vi "Split Registers by Direction.vi"(7 "Group":bool, 8 "error in":errorcluster, 11 "vi info":T2 {"RegisterMap"."Address" format="%.0x"}) -> (0 "error out":errorcluster, 1 "FXP channels out":T1(array[cluster]), 2 "Controls":T9[](array[typedef]) {"Data Type" format="%.0x"}, 3 "Indicator":T9[](array[typedef]) {"Data Type" format="%.0x"})   [LabVIEW 2018, in "FPGA Addon System Explorer.lvlib"]
uses:
  FPGA Addon System Explorer.lvlib
  Addon Shared/Types/Register Information.ctl
  Addon Shared/Types/Data Type.ctl
  <vilib>/rvi/Bitfile/niFpgaBitfileStructure_VI.ctl
  <vilib>/rvi/Bitfile/nirviControlStructure.ctl
  <vilib>/rvi/Bitfile/nirviTypdefDescription.ctl
  <vilib>/rvi/Bitfile/nirviMechanicalAction.ctl
  <vilib>/rvi/Bitfile/nirviSubControlStructure.ctl
  <vilib>/rvi/Bitfile/nirviClusterElementControl.ctl
  <vilib>/picture/picture.llb/imagedata.ctl
  Submodules/Source/Types/PWM.Measure.Analog.Measurement.ctl
  Submodules/Source/Types/PWM.Measure.Digital.Measurement.ctl
  Submodules/Source/Types/Static.Measure.Digital.Measurement.ctl
  Submodules/Source/Types/QuadratureEncoder.Measure.Digital.Measurement.ctl
  Submodules/Source/Types/PWM.Generate.Digital.Settings.ctl
  Submodules/Source/Types/PWM.Measure.Analog.Settings.ctl
  Submodules/Source/Types/PWM.Measure.Digital.Settings.ctl
  Submodules/Source/Types/Sine.Generate.Settings.ctl
  Submodules/Source/Types/Static.Generate.Digital.Settings.ctl
  Submodules/Source/Types/Static.Measure.Digital.Settings.ctl
  Submodules/Source/Types/WSS.Generate.Digital.Settings.ctl
  Submodules/Source/Types/QuadratureEncoder.Measure.Digital.Settings.ctl
  Addon Shared/FPGA Addon Shared.lvlib
  Submodules/Source/Speciality FPGA IO.lvlib
  <vilib>/Utility/Data Type/NI_Data Type.lvlib
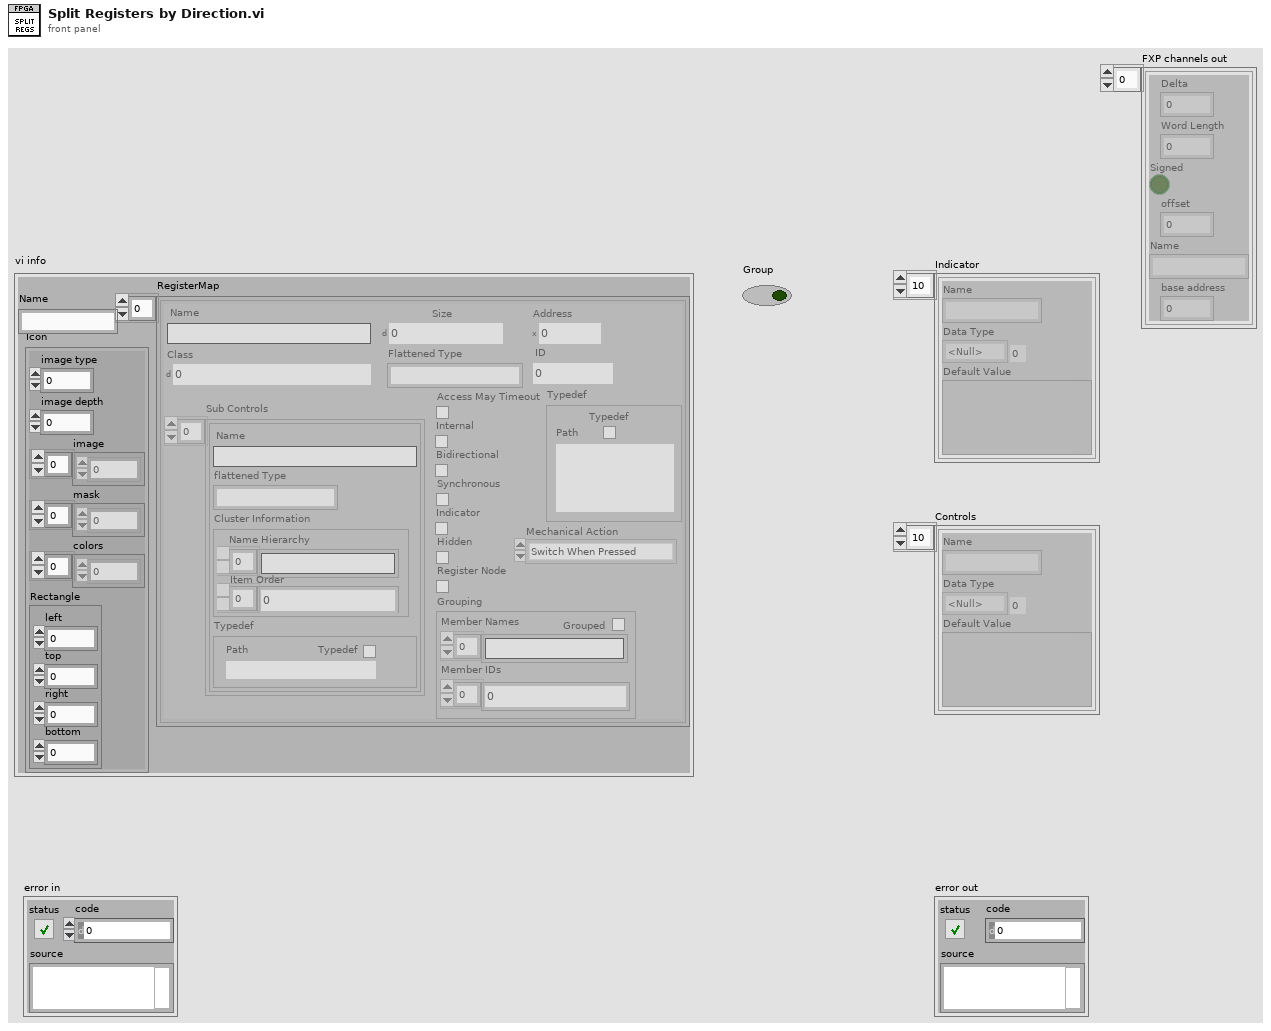
[diagram p1: front panel]
types:
  T1 = cluster{"Delta":dbl, "Word Length":i8, "Signed":bool, "offset":i32, "Name":string, "base address":i32}[]
  T2 = typedef "niFpgaBitfileStructure_VI.ctl" = cluster{"Name":string, "RegisterMap":T3[], "Icon":T8}
  T3 = typedef "nirviControlStructure.ctl" = cluster{"Name":string, "Hidden":bool, "Indicator":bool, "Flattened Type":string, "Grouping":cluster{"Grouped":bool, "Member Names":string[], "Member IDs":u32[]}, "Address":u32, "Size":u32, "Class":u32, "Internal":bool, "Typedef":T4, "ID":u32, "Bidirectional":bool, "Synchronous":bool, "Mechanical Action":T5, "Sub Controls":T6[], "Access May Timeout":bool, "Register Node":bool}
  T4 = typedef "nirviTypdefDescription.ctl" = cluster{"Typedef":bool, "Path":path}
  T5 = typedef "nirviMechanicalAction.ctl" = enum8{"Switch When Pressed", "Switch When Released", "Switch Until Released", "Latch When Pressed", "Latch When Released", "Latch Until Released"}
  T6 = typedef "nirviSubControlStructure.ctl" = cluster{"Name":string, "flattened Type":string, "Cluster Information":T7, "Typedef":T4}
  T7 = typedef "nirviClusterElementControl.ctl" = cluster{"Name Hierarchy":string[], "Item Order":u32[]}
  T8 = typedef "imagedata.ctl" = cluster{"image type":i32, "image depth":i32, "image":u8[], "mask":u8[], "colors":u32[], "Rectangle":cluster{"left":i16, "top":i16, "right":i16, "bottom":i16}}
  T9 = typedef "FPGA Addon Shared.lvlib/Register Information.ctl" = cluster{"Name":string, "Data Type":T10, "Default Value":variant}
  T10 = typedef "FPGA Addon Shared.lvlib/Data Type.ctl" = enum8{"<Null>", "I8", "I16", "I32", "I64", "U8", "U16", "U32", "U64", "SGL", "Boolean", "Analog PWM In Settings", "Analog PWM In", "Digital PWM In Settings", "Digital PWM In", "Digital PWM Out", "Sine Out", "FXP+/-24.5", "FXP+/-16.5", "FXP+/-32.8", "FXP+/-64.32", "FXP+/-16.7", "FXP+/-20.5", "FXP+/-27.5", "FXP+/-32.16", "FXP+16.3", "FXP+18.3", "Digital Static In", "Digital Static Out", "Digital Static In Settings", "Digital WSS Out", "Quad Encoder Settings", "Quad Encoder In", "Group"}
  T11 = typedef "Speciality FPGA IO.lvlib/QuadratureEncoder.Measure.Digital.Measurement.ctl" = cluster{"POSITION":i32}
  T12 = typedef "Speciality FPGA IO.lvlib/Static.Measure.Digital.Measurement.ctl" = cluster{"STATE":bool}
  T13 = typedef "Speciality FPGA IO.lvlib/PWM.Measure.Digital.Measurement.ctl" = cluster{"ACTIVE TICKS":u32, "INACTIVE TICKS":u32, "ACQ TICKS":u32}
  T14 = typedef "Speciality FPGA IO.lvlib/PWM.Measure.Analog.Measurement.ctl" = cluster{"ACTIVE TICKS":u32, "INACTIVE TICKS":u32, "ACQ TICKS":u32, "ACTIVE VOLTAGE":fxp<+/-,32,8>, "INACTIVE VOLTAGE":fxp<+/-,32,8>}
  T15 = typedef "Speciality FPGA IO.lvlib/QuadratureEncoder.Measure.Digital.Settings.ctl" = cluster{"DIRECTION":u8, "RESET VALUE":i32, "A RESET STATE":bool, "B RESET STATE":bool, "Z RESET STATE":bool}
  T16 = typedef "Speciality FPGA IO.lvlib/WSS.Generate.Digital.Settings.ctl" = cluster{"ACTIVE EDGE":bool, "ACTIVE TICKS":u32, "INACTIVE TICKS":u32, "DATA":u8, "SENSOR TYPE":u8}
  T17 = typedef "Speciality FPGA IO.lvlib/Static.Measure.Digital.Settings.ctl" = cluster{"ACTIVE EDGE":bool}
  T18 = typedef "Speciality FPGA IO.lvlib/Static.Generate.Digital.Settings.ctl" = cluster{"ACTIVE EDGE":bool, "OUTPUT":bool}
  T19 = typedef "Speciality FPGA IO.lvlib/Sine.Generate.Settings.ctl" = cluster{"AMP":fxp<+/-,32,8>, "OFFSET":fxp<+/-,32,8>, "PERIODS/TICKS":fxp<+,32,0>}
  T20 = typedef "Speciality FPGA IO.lvlib/PWM.Measure.Digital.Settings.ctl" = cluster{"ACTIVE EDGE":bool, "TIMEOUT":u32}
  T21 = typedef "Speciality FPGA IO.lvlib/PWM.Measure.Analog.Settings.ctl" = cluster{"ACTIVE EDGE":bool, "TIMEOUT":u32, "THRESHOLD":fxp<+/-,32,8>}
  T22 = typedef "Speciality FPGA IO.lvlib/PWM.Generate.Digital.Settings.ctl" = cluster{"ACTIVE EDGE":bool, "ACTIVE TICKS":u32, "INACTIVE TICKS":u32}
  T23 = cluster{"Delta":dbl, "Word Length":i8, "Signed":bool, "offset":i32, "Name":string, "base address":i32}
  T24 = typedef "Type Descriptor Enumeration__ogtk.ctl" = enum8{"<Null>", "I8", "I16", "I32", "I64", "U8", "U16", "U32", "U64", "SGL", "DBL", "EXT", "CSG", "CDB", "CXT", "0x0F", "0x10", "0x11", "0x12", "0x13", "0x14", "Enum U8", "Enum U16", "Enum U32", "Enum U64", "SGL PQ", "DBL PQ", "EXT PQ", "CSG PQ", "CDB PQ", "CXT PQ", "0x1F", "0x20", "Boolean", "0x22", "0x23", "0x24", "0x25", "0x26", "0x27", "0x28", "0x29", "0x2A", "0x2B", "0x2C", "0x2D", "0x2E", "0x2F", "String", "0x31", "Path", "Pict", "0x34", "0x35", "0x36", "DAQ", "0x38", "0x39", "0x3A", "0x3B", "0x3C", "0x3D", "0x3E", "0x3F", "Array", "0x41", "0x42", "0x43", "0x44", "0x45", "0x46", "0x47", "0x48", "0x49", "0x4A", "0x4B", "0x4C", "0x4D", "0x4E", "0x4F", "Cluster", "0x51", "0x52", "Variant", "Waveform", "0x55", "0x56", "0x57", "0x58", "0x59", "0x5A", "0x5B", "0x5C", "0x5D", "0x5E", "0x5F", "0x60", "0x61", "0x62", "0x63", "0x64", "0x65", "0x66", "0x67", "0x68", "0x69", "0x6A", "0x6B", "0x6C", "0x6D", "0x6E", "0x6F", "Refnum"}
  T25 = typedef "LVFixedPointRepBitsTypeDef.ctl" = cluster{"Signed":bool, "Word Length":u32, "Integer Word Length":i32}
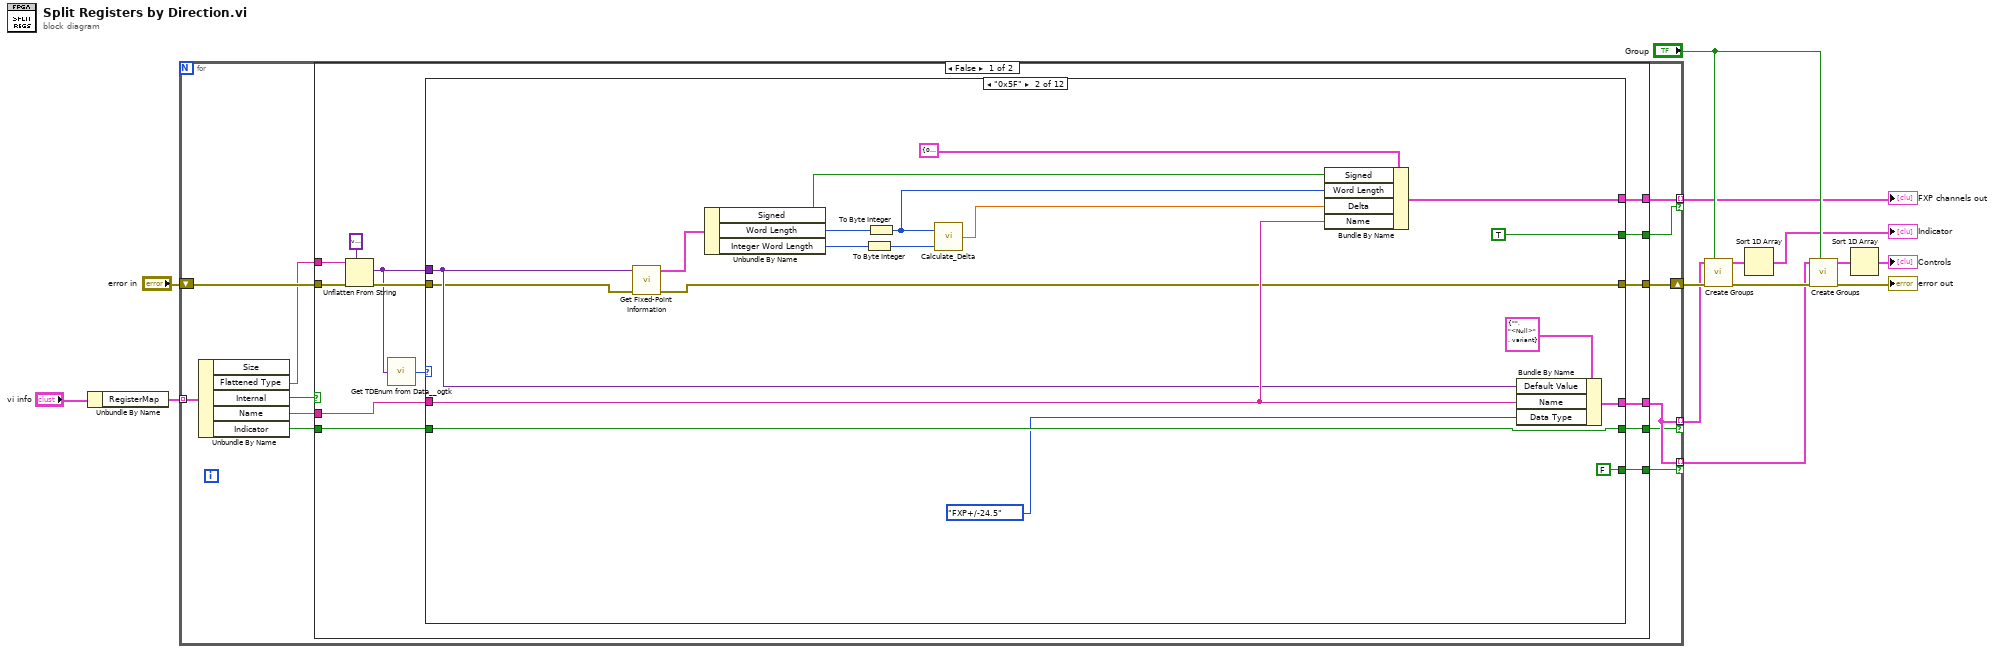
[diagram p0: block diagram]
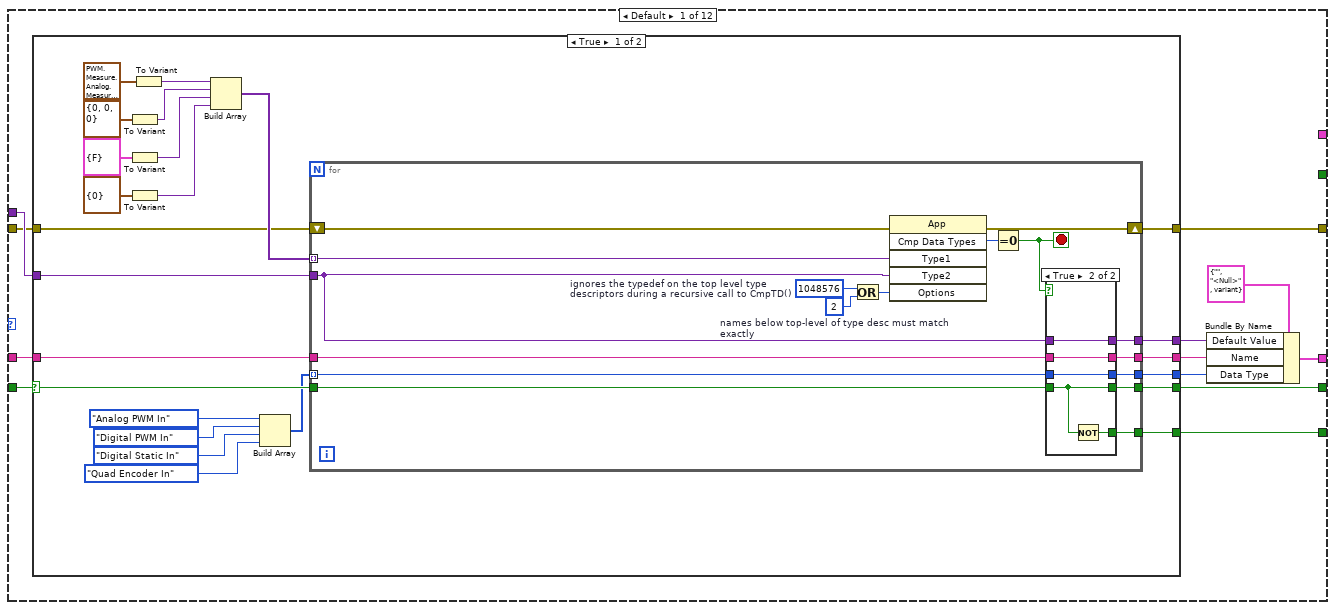
[diagram p2: hidden frame]
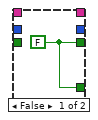
[diagram p3: hidden frame]
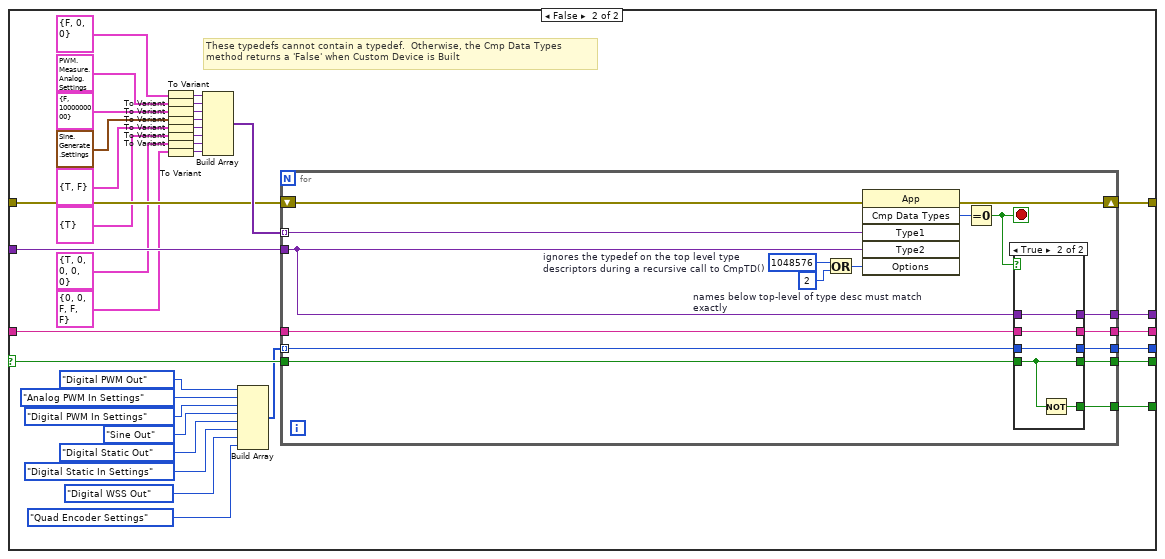
[diagram p4: hidden frame]
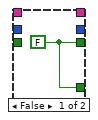
[diagram p5: hidden frame]
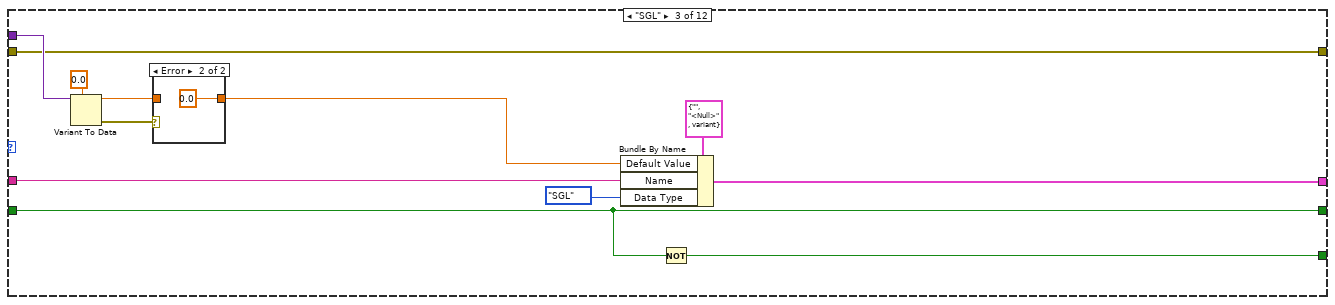
[diagram p6: hidden frame]
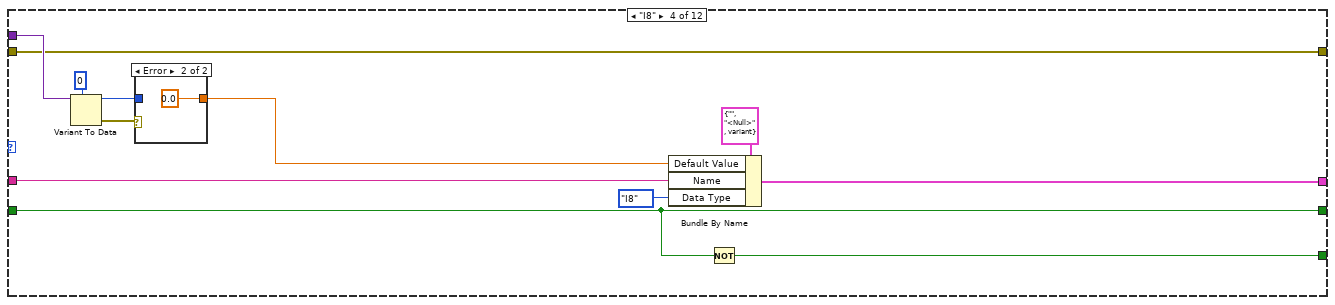
[diagram p8: hidden frame]
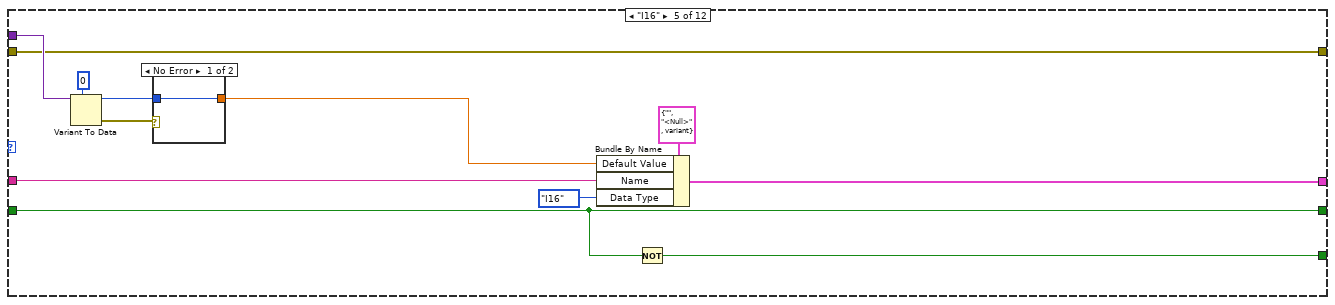
[diagram p10: hidden frame]
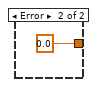
[diagram p11: hidden frame]
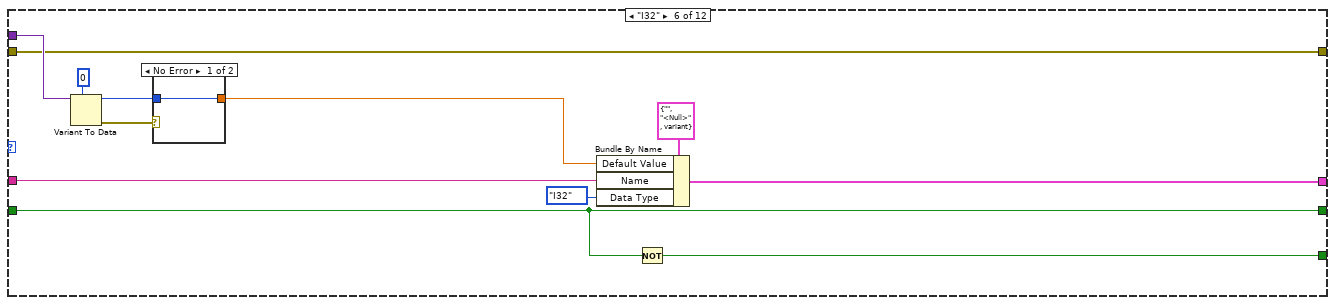
[diagram p12: hidden frame]
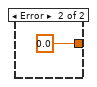
[diagram p13: hidden frame]
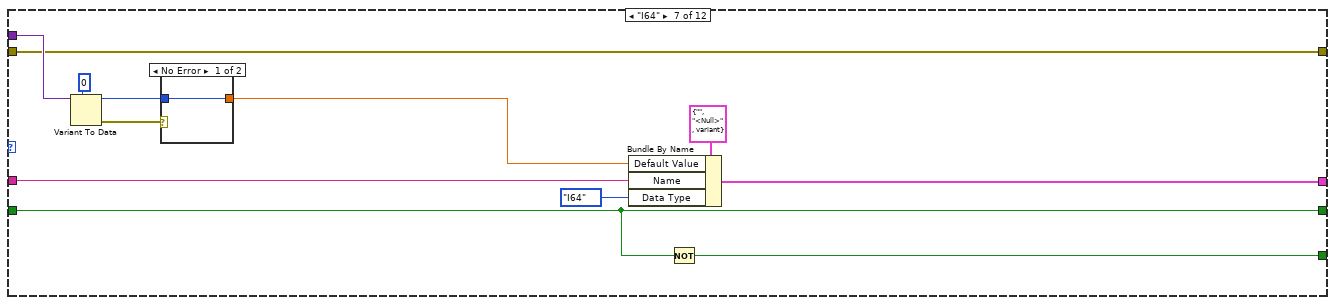
[diagram p14: hidden frame]
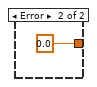
[diagram p15: hidden frame]
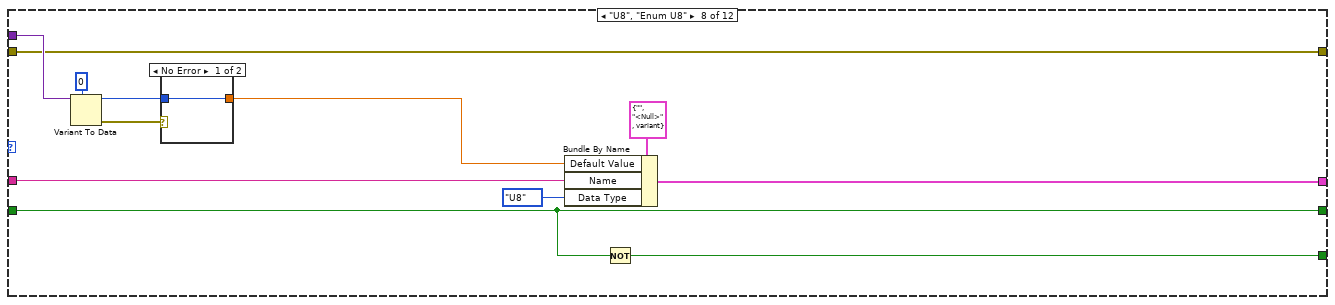
[diagram p16: hidden frame]
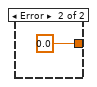
[diagram p17: hidden frame]
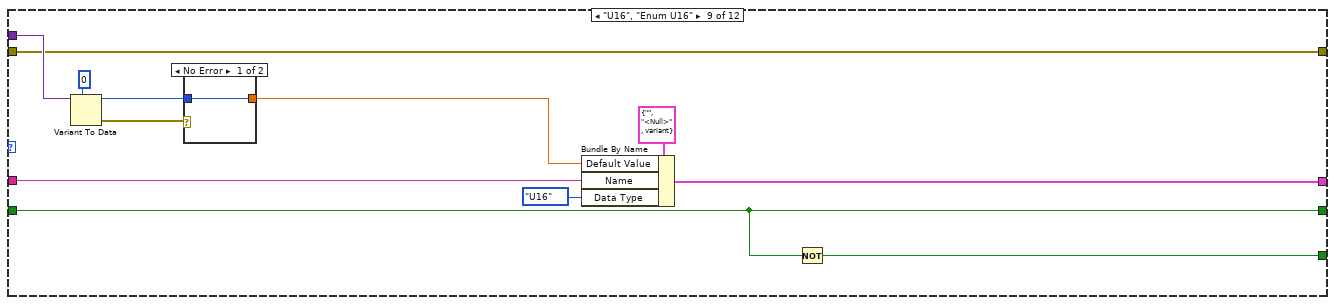
[diagram p18: hidden frame]
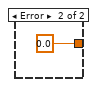
[diagram p19: hidden frame]
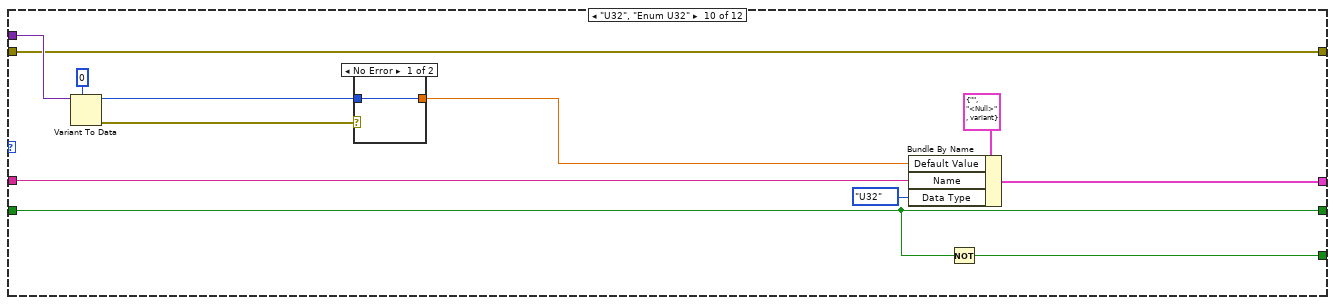
[diagram p20: hidden frame]
diagram:
  n1 = Unbundle By Name("vi info") -> ("RegisterMap"=w14:T3[])
  n2 = for {
    tunnel: w14 -> [w21] mode=indexing
    tunnel: [w26] -> w7 mode=indexing if=w25
    tunnel: [w26] -> w6 mode=indexing if=w24
    shift-right: [w23] -> w11
    shift-left: "error in" -> [w22]
    tunnel: [w16] -> w1 mode=indexing if=w15
    n3 = Unbundle By Name(w21) -> ("Flattened Type"=w17:string, "Internal"=w18:bool, "Name"=w19:string, "Indicator"=w20:bool)  [unwired: 1 out]
    n4 = case shown="False" w18 {
      tunnel: w19 -> [w39 _]
      tunnel: w20 -> [w38 _]
      tunnel: [w37 _] -> w26
      tunnel: [w36 w320] -> w25
      tunnel: [w35 w320] -> w24
      tunnel: w17 -> [w32 _]
      tunnel: [w34 w319] -> w23
      tunnel: w22 -> [w31 w319]
      tunnel: [w28 _] -> w16
      tunnel: [w27 _] -> w15
      frame False {
        n5 = Unflatten From String(type=variant ("Variant"), binary string=w32, error in (no error)=w31) -> (value=w29:variant, error out=w30:errorcluster)  [unwired: 3 out]
        n6 = call <userlib>:"Get TDEnum from Data__ogtk.vi"("Data"=w29) -> ("Type Descriptor Enumeration"=w40:T24)  [unwired: 4 in]
        n7 = case shown="\"0x5F\"" w40 {
          tunnel: [w52 w174 w186 w200 w214 w228 w242 w256 w270 w284 w298 w312] -> w36
          tunnel: w38 -> [w47 w174 w186 w200 w214 w228 w242 w256 w270 w284 w298 w312]
          tunnel: w39 -> [w48 w175 w188 w202 w216 w230 w244 w258 w272 w286 w300 w314]
          tunnel: [w49 w176 w187 w201 w215 w229 w243 w257 w271 w285 w299 w313] -> w37
          tunnel: [w51 FALSE ("Boolean") w185 w199 w213 w227 w241 w255 w269 w283 w297 w311] -> w35
          tunnel: w29 -> [w46 w173 w184 w198 w212 w226 w240 w254 w268 w282 w296 w310]
          tunnel: [w42 w165 w178 w192 w206 w220 w234 w248 w262 w276 w290 w304] -> w34
          tunnel: w30 -> [w41 w166 w178 w192 w206 w220 w234 w248 w262 w276 w290 w304]
          tunnel: [_ w169 _ _ _ _ _ _ _ _ _ _] -> w28
          tunnel: [_ TRUE _ _ _ _ _ _ _ _ _ _] -> w27
          frame Default {
            n8 = case shown="True" w47 {
              selector: w47 -> [w71 w131]
              tunnel: [w76 w135] -> w52
              tunnel: [w75 w134] -> w51
              tunnel: w48 -> [w74 w133]
              tunnel: w46 -> [w65 w127]
              tunnel: [w64 w126] -> w45
              tunnel: [w63 w125] -> w44
              tunnel: [w62 w124] -> w43
              tunnel: [w60 w115] -> w42
              tunnel: w41 -> [w59 w116]
              frame True {
                n9 = To Variant(anything=T13 {"ACTIVE TICKS"=0, "INACTIVE TICKS"=0, "ACQ TICKS"=0} ("Cached.Data")) -> (Variant=w69:variant)
                n10 = To Variant(anything=T12 {"STATE"=FALSE} ("Cached.Data")) -> (Variant=w57:variant)
                n11 = To Variant(anything=T11 {"POSITION"=0} ("Cached.Data")) -> (Variant=w53:variant)
                n12 = To Variant(anything=T14 {"ACTIVE TICKS"=0, "INACTIVE TICKS"=0, "ACQ TICKS"=0, "ACTIVE VOLTAGE"=0.0, "INACTIVE VOLTAGE"=0.0} ("Cached.Data")) -> (Variant=w70:variant)
                n13 = Build Array(w70, w69, w57, w53) -> (w66:variant[])
                n14 = Build Array(Data_Type."Analog PWM In" ("Data Type"), Data_Type."Digital PWM In" ("Data Type"), Data_Type."Digital Static In" ("Data Type"), Data_Type."Quad Encoder In" ("Data Type")) -> (w61:T10[])
                n15 = for {
                  tunnel: w65 -> [w80]
                  tunnel: [w91] -> w75
                  tunnel: w74 -> [w90]
                  tunnel: w66 -> [w82] mode=indexing
                  tunnel: [w89] -> w63
                  tunnel: [w88] -> w64
                  tunnel: [w87] -> w62
                  tunnel: w61 -> [w86] mode=indexing
                  tunnel: w71 -> [w93]
                  tunnel: [w92] -> w76
                  shift-right: [w77] -> w60
                  shift-left: w59 -> [w78]
                  stop <- w81 stop-if-true
                  w79 = 2  # names below top-level of type desc must match exactly
                  w84 = 1048576  # ignores the typedef on the top level type descriptors during a recursive call to CmpTD()
                  n16 = Or(x=w84, y=w79) -> (x .or. y?=w85:i32)
                  n17 = invoke class="App" method="Cmp Data Types"(error in=w78, "Type1"=w82, "Type2"=w80, "Options"=w85) -> (error out=w77:errorcluster, "Compare Data Types"=w83:i32)  [unwired: 2 in, 4 out]
                  n18 = Equal To 0?(x=w83) -> (x = 0?=w81:bool)
                  n19 = case shown="True" w81 {
                    tunnel: w93 -> [_ w99]
                    tunnel: [w94 w99] -> w92
                    tunnel: [w94 w98] -> w91
                    tunnel: w90 -> [_ w96]
                    tunnel: [_ w97] -> w89
                    tunnel: w80 -> [_ w97]
                    tunnel: [_ w96] -> w88
                    tunnel: [_ w95] -> w87
                    tunnel: w86 -> [_ w95]
                    frame False {
                      w94 = FALSE ("Boolean")
                    }
                    frame True {
                      n20 = Not(x=w99) -> (.not. x?=w98:bool)
                    }
                  }
                }
              }
              frame False {
                # "These typedefs cannot contain a typedef.  Otherwise, the Cmp Data Types \nmethod returns a 'False' when Custom Device is Built"
                n21 = To Variant(anything=T22 {"ACTIVE EDGE"=FALSE, "ACTIVE TICKS"=0, "INACTIVE TICKS"=0} ("Channel.Settings")) -> (Variant=w130:variant)
                n22 = To Variant(anything=T21 {"ACTIVE EDGE"=FALSE, "TIMEOUT"=1000000000, "THRESHOLD"=3.0} ("Channel.Settings")) -> (Variant=w120:variant)
                n23 = To Variant(anything=T20 {"ACTIVE EDGE"=FALSE, "TIMEOUT"=1000000000} ("Channel.Settings")) -> (Variant=w119:variant)
                n24 = To Variant(anything=T19 {"AMP"=0.0, "OFFSET"=0.0, "PERIODS/TICKS"=0.0002500000409781933} ("Settings")) -> (Variant=w113:variant)
                n25 = To Variant(anything=T18 {"ACTIVE EDGE"=TRUE, "OUTPUT"=FALSE} ("Settings")) -> (Variant=w111:variant)
                n26 = To Variant(anything=T17 {"ACTIVE EDGE"=TRUE} ("Settings")) -> (Variant=w108:variant)
                n27 = To Variant(anything=T16 {"ACTIVE EDGE"=TRUE, "ACTIVE TICKS"=0, "INACTIVE TICKS"=0, "DATA"=0, "SENSOR TYPE"=0} ("Wheel Speed Sensor Settings")) -> (Variant=w104:variant)
                n28 = To Variant(anything=T15 {"DIRECTION"=0, "RESET VALUE"=0, "A RESET STATE"=FALSE, "B RESET STATE"=FALSE, "Z RESET STATE"=FALSE} ("Settings")) -> (Variant=w101:variant)
                n29 = Build Array(w130, w120, w119, w113, w111, w108, w104, w101) -> (w128:variant[])
                n30 = Build Array(Data_Type."Digital PWM Out" ("Data Type"), Data_Type."Analog PWM In Settings" ("Data Type"), Data_Type."Digital PWM In Settings" ("Data Type"), Data_Type."Sine Out" ("Data Type"), Data_Type."Digital Static Out" ("Data Type"), Data_Type."Digital Static In Settings" ("Data Type"), Data_Type."Digital WSS Out" ("Data Type"), Data_Type."Quad Encoder Settings" ("Data Type")) -> (w123:T10[])
                n31 = for {
                  tunnel: w127 -> [w141]
                  tunnel: [w150] -> w134
                  tunnel: w133 -> [w149]
                  tunnel: w128 -> [w140] mode=indexing
                  tunnel: [w148] -> w125
                  tunnel: [w147] -> w126
                  tunnel: [w146] -> w124
                  tunnel: w123 -> [w145] mode=indexing
                  tunnel: w131 -> [w152]
                  tunnel: [w151] -> w135
                  shift-right: [w136] -> w115
                  shift-left: w116 -> [w137]
                  stop <- w138 stop-if-true
                  w143 = 2  # names below top-level of type desc must match exactly
                  w142 = 1048576  # ignores the typedef on the top level type descriptors during a recursive call to CmpTD()
                  n32 = Or(x=w142, y=w143) -> (x .or. y?=w144:i32)
                  n33 = invoke class="App" method="Cmp Data Types"(error in=w137, "Type1"=w140, "Type2"=w141, "Options"=w144) -> (error out=w136:errorcluster, "Compare Data Types"=w139:i32)  [unwired: 2 in, 4 out]
                  n34 = Equal To 0?(x=w139) -> (x = 0?=w138:bool)
                  n35 = case shown="True" w138 {
                    tunnel: w152 -> [_ w158]
                    tunnel: [w153 w158] -> w151
                    tunnel: [w153 w157] -> w150
                    tunnel: w149 -> [_ w155]
                    tunnel: [_ w156] -> w148
                    tunnel: w141 -> [_ w156]
                    tunnel: [_ w155] -> w147
                    tunnel: [_ w154] -> w146
                    tunnel: w145 -> [_ w154]
                    frame False {
                      w153 = FALSE ("Boolean")
                    }
                    frame True {
                      n36 = Not(x=w158) -> (.not. x?=w157:bool)
                    }
                  }
                }
              }
            }
            n37 = Bundle By Name(cluster=T9 {"Name"="", "Data Type"=enum."<Null>", "Default Value"=variant(refnum<class> refnum)}, "Default Value"=w44, "Name"=w45, "Data Type"=w43) -> (w49:T9)
          }
          frame "0x5F" {
            n38 = call <vilib>:"Get Fixed-Point Information.vi"("error in (no error)"=w166, "Variant"=w173) -> ("error out"=w165:errorcluster, "FXP Representation"=w171:T25)  [unwired: 6 in, 2 out]
            n39 = Unbundle By Name(w171) -> ("Signed"=w170:bool, "Word Length"=w162:u32, "Integer Word Length"=w164:i32)
            n40 = To Byte Integer(number=w164) -> (8bit integer=w163:i8)
            n41 = To Byte Integer(number=w162) -> (8bit integer=w160:i8)
            n42 = call "Calculate_Delta.vi"("WordLength"=w163, "IntegerWordLength"=w160) -> ("delta"=w161:dbl)
            n43 = Bundle By Name(cluster=T23 {"Delta"=0.0, "Word Length"=0, "Signed"=FALSE, "offset"=0, "Name"="", "base address"=0}, "Signed"=w170, "Word Length"=w160, "Delta"=w161, "Name"=w175) -> (w169:T23)
            n44 = Bundle By Name(cluster=T9 {"Name"="", "Data Type"=enum."<Null>", "Default Value"=variant(refnum<class> refnum)}, "Default Value"=w173, "Name"=w175, "Data Type"=Data_Type."FXP+/-24.5") -> (w176:T9)
          }
          frame "SGL" {
            n45 = Variant To Data(type=sgl 0.0, Variant=w184) -> (data=w180:sgl, error out=w182:errorcluster)  [unwired: 1 in]
            n46 = case shown="Error" w182 {
              tunnel: [w190 0.0] -> w181
              tunnel: w180 -> [w190 _]
              frame No Error {
              }
              frame Error {
              }
            }
            n47 = Bundle By Name(cluster=T9 {"Name"="", "Data Type"=enum."<Null>", "Default Value"=variant(refnum<class> refnum)}, "Default Value"=w181, "Name"=w188, "Data Type"=Data_Type."SGL") -> (w187:T9)
            n48 = Not(x=w186) -> (.not. x?=w185:bool)
          }
          frame "I8" {
            n49 = Variant To Data(type=i8 0, Variant=w198) -> (data=w194:i8, error out=w196:errorcluster)  [unwired: 1 in]
            n50 = case shown="Error" w196 {
              tunnel: [w204 0.0] -> w195
              tunnel: w194 -> [w204 _]
              frame No Error {
              }
              frame Error {
              }
            }
            n51 = Bundle By Name(cluster=T9 {"Name"="", "Data Type"=enum."<Null>", "Default Value"=variant(refnum<class> refnum)}, "Default Value"=w195, "Name"=w202, "Data Type"=Data_Type."I8") -> (w201:T9)
            n52 = Not(x=w200) -> (.not. x?=w199:bool)
          }
          frame "I16" {
            n53 = Variant To Data(type=i16 0, Variant=w212) -> (data=w208:i16, error out=w210:errorcluster)  [unwired: 1 in]
            n54 = case shown="No Error" w210 {
              tunnel: [w218 0.0] -> w209
              tunnel: w208 -> [w218 _]
              frame No Error {
              }
              frame Error {
              }
            }
            n55 = Bundle By Name(cluster=T9 {"Name"="", "Data Type"=enum."<Null>", "Default Value"=variant(refnum<class> refnum)}, "Default Value"=w209, "Name"=w216, "Data Type"=Data_Type."I16") -> (w215:T9)
            n56 = Not(x=w214) -> (.not. x?=w213:bool)
          }
          frame "I32" {
            n57 = Variant To Data(type=0, Variant=w226) -> (data=w222:i32, error out=w224:errorcluster)  [unwired: 1 in]
            n58 = case shown="No Error" w224 {
              tunnel: [w232 0.0] -> w223
              tunnel: w222 -> [w232 _]
              frame No Error {
              }
              frame Error {
              }
            }
            n59 = Bundle By Name(cluster=T9 {"Name"="", "Data Type"=enum."<Null>", "Default Value"=variant(refnum<class> refnum)}, "Default Value"=w223, "Name"=w230, "Data Type"=Data_Type."I32") -> (w229:T9)
            n60 = Not(x=w228) -> (.not. x?=w227:bool)
          }
          frame "I64" {
            n61 = Variant To Data(type=i64 0, Variant=w240) -> (data=w236:i64, error out=w238:errorcluster)  [unwired: 1 in]
            n62 = case shown="No Error" w238 {
              tunnel: [w246 0.0] -> w237
              tunnel: w236 -> [w246 _]
              frame No Error {
              }
              frame Error {
              }
            }
            n63 = Bundle By Name(cluster=T9 {"Name"="", "Data Type"=enum."<Null>", "Default Value"=variant(refnum<class> refnum)}, "Default Value"=w237, "Name"=w244, "Data Type"=Data_Type."I64") -> (w243:T9)
            n64 = Not(x=w242) -> (.not. x?=w241:bool)
          }
          frame "U8", "Enum U8" {
            n65 = Variant To Data(type=u8 0, Variant=w254) -> (data=w250:u8, error out=w252:errorcluster)  [unwired: 1 in]
            n66 = case shown="No Error" w252 {
              tunnel: [w260 0.0] -> w251
              tunnel: w250 -> [w260 _]
              frame No Error {
              }
              frame Error {
              }
            }
            n67 = Bundle By Name(cluster=T9 {"Name"="", "Data Type"=enum."<Null>", "Default Value"=variant(refnum<class> refnum)}, "Default Value"=w251, "Name"=w258, "Data Type"=Data_Type."U8") -> (w257:T9)
            n68 = Not(x=w256) -> (.not. x?=w255:bool)
          }
          frame "U16", "Enum U16" {
            n69 = Variant To Data(type=u16 0, Variant=w268) -> (data=w264:u16, error out=w266:errorcluster)  [unwired: 1 in]
            n70 = case shown="No Error" w266 {
              tunnel: [w274 0.0] -> w265
              tunnel: w264 -> [w274 _]
              frame No Error {
              }
              frame Error {
              }
            }
            n71 = Bundle By Name(cluster=T9 {"Name"="", "Data Type"=enum."<Null>", "Default Value"=variant(refnum<class> refnum)}, "Default Value"=w265, "Name"=w272, "Data Type"=Data_Type."U16") -> (w271:T9)
            n72 = Not(x=w270) -> (.not. x?=w269:bool)
          }
          frame "U32", "Enum U32" {
            n73 = Variant To Data(type=u32 0, Variant=w282) -> (data=w278:u32, error out=w280:errorcluster)  [unwired: 1 in]
            n74 = case shown="No Error" w280 {
              tunnel: [w288 0.0] -> w279
              tunnel: w278 -> [w288 _]
              frame No Error {
              }
              frame Error {
              }
            }
            n75 = Bundle By Name(cluster=T9 {"Name"="", "Data Type"=enum."<Null>", "Default Value"=variant(refnum<class> refnum)}, "Default Value"=w279, "Name"=w286, "Data Type"=Data_Type."U32") -> (w285:T9)
            n76 = Not(x=w284) -> (.not. x?=w283:bool)
          }
          frame "U64", "Enum U64" {
            n77 = Variant To Data(type=u64 0, Variant=w296) -> (data=w292:u64, error out=w294:errorcluster)  [unwired: 1 in]
            n78 = case shown="No Error" w294 {
              tunnel: [w302 0.0] -> w293
              tunnel: w292 -> [w302 _]
              frame No Error {
              }
              frame Error {
              }
            }
            n79 = Bundle By Name(cluster=T9 {"Name"="", "Data Type"=enum."<Null>", "Default Value"=variant(refnum<class> refnum)}, "Default Value"=w293, "Name"=w300, "Data Type"=Data_Type."U64") -> (w299:T9)
            n80 = Not(x=w298) -> (.not. x?=w297:bool)
          }
          frame "Boolean" {
            n81 = Variant To Data(type=FALSE, Variant=w310) -> (data=w306:bool, error out=w308:errorcluster)  [unwired: 1 in]
            n82 = case shown="No Error" w308 {
              tunnel: [w316 0.0] -> w307
              tunnel: w306 -> [w317 _]
              frame No Error {
                n83 = Boolean To (0,1)(Boolean=w317) -> (0, 1=w316:i16)
              }
              frame Error {
              }
            }
            n84 = Bundle By Name(cluster=T9 {"Name"="", "Data Type"=enum."<Null>", "Default Value"=variant(refnum<class> refnum)}, "Default Value"=w307, "Name"=w314, "Data Type"=Data_Type."Boolean") -> (w313:T9)
            n85 = Not(x=w312) -> (.not. x?=w311:bool)
          }
        }
      }
      frame True {
        w320 = FALSE ("Boolean")
      }
    }
  }
  "FXP channels out" <- w1
  n86 = call "Create Groups.vi"("Group"="Group", "error in (no error)"=w11, "Channels"=w7) -> ("error out"=w10:errorcluster, "Channels out"=w5:T9[])  [unwired: 7 in]
  n87 = Sort 1D Array(array=w5) -> (sorted array=→"Indicator":T9[])
  n88 = call "Create Groups.vi"("Group"="Group", "error in (no error)"=w10, "Channels"=w6) -> ("error out"=→"error out":errorcluster, "Channels out"=w3:T9[])  [unwired: 7 in]
  n89 = Sort 1D Array(array=w3) -> (sorted array=→"Controls":T9[])
